vi "RTG Example.vi"() -> ()   [LabVIEW 2020, in "RTG Examples.lvlib"]
doc: "This example illustrates how to use the RTG local API to control the RTG."
uses:
  RTG Examples.lvlib
  <vilib>/RTG/API/ip/common/host-types/Target Configuration.ctl
  <vilib>/RTG/API/ip/common/host-types/Synchronization - Host.ctl
  <vilib>/RTG/API/ip/common/host-types/Synchronization Mode - Host.ctl
  <vilib>/RTG/API/ip/common/host-types/Basic Target - Host.ctl
  <vilib>/RTG/API/interface/public/State.ctl
  <vilib>/RTG/coprocessor/host/RTG Coprocessor Link Interface/Public/Coprocessor Status.ctl
  <vilib>/RTG/API/ip/common/host-types/Target Motion Parameters.ctl
  <vilib>/RTG/API/ip/common/host-types/Single Target Motion Parameters.ctl
  support/Options - API Mode.ctl
  support/Options - Calibration.ctl
  support/Options - Remote.ctl
  <vilib>/RTG/API/interface/public/Coprocessor Link Status.ctl
  <vilib>/Utility/error.llb/Error Cluster From Error Code.vi
  <vilib>/rvi/errors/niLvFpgaAdjustHostInterfaceError.vi
  <vilib>/rvi/interface/nirviReadWriteControl/nirviReadWriteControl.xnode
  <vilib>/RTG/API/interface/NI-RTG Interface.lvclass
  <vilib>/RTG/coprocessor/host/RTG Coprocessor Link Interface/RTG Coprocessor Link Interface.lvclass
  <vilib>/RTG/API/ip/common/host-types/Host Data Types v1.lvlib
  NiFpgaLv.dll
  <vilib>/rvi/interface/Simulation/niFpgaSimulationCallBeginRW.vi
panel:
  out "Bitfiles Loaded":bool
  out "RTG Status":string
  out "RTG State":T1
  in  "tab":T2(tab)
  in  "abort system self cal":bool
  in  "Set PRIs":bool
  in  "PRI (s)":dbl[](array[numeric]) format="%#_6p"
  in  "Calibrate":bool=TRUE
  in  "Instrument Names":string[](array[string])=["5831_0"]
  in  "Center Freqeuncies (Hz)":dbl[](array[numeric])=[5500000000.0] format="%#_6p"
  in  "Reference Levels (dBm)":dbl[](array[numeric])=[0.0]
  in  "mmWave Radio Heads Enable":bool[](array[boolean])
  in  "External Delay (s)":dbl[](array[numeric]) format="%#_6p"
  in  "External Attenuations (dB)":dbl[](array[numeric])
  in  "Offset Frequencies (Hz)":dbl[](array[numeric]) format="%#_6p"
  out "Error Out":errorcluster caption="error out"
  in  "RTG API Options":T6={"API Mode"=enum."Local", "Calibration Options"={"enable internal loopback  "=FALSE, "enable overwrite cal data  "=FALSE, "enable save cal data           "=FALSE, "disable self cal range          "=FALSE}, "Remote Options"={"ip address"="", "port"="50052", "certificate path"=path "", "timeout (ms)"=15000}, "ini file path"=path ""}
  in  "Option String Override":string
  in  "Coprocessor Names":string[](array[string])
  out "Versions":string[](array[string])
  out "Max Common Attenuations (dB)":dbl[](array[numeric])
  out "Min Common Attenuations (dB)":dbl[](array[numeric])
  out "Min Latencies (s)":dbl[](array[numeric]) format="%#_6p"
  in  "configure common attenuation":bool
  in  "Common Attenuation (dB)":dbl
  in  "set hardware trigger":bool
  in  "send target motion":bool
  in  "Auto Send Software Trigger":bool
  in  "Prepend Software Trigger":bool
  in  "send files":bool
  in  "Target Configuration Files":path[](array[path])
  in  "pulse detection calibration":bool
  in  "send target config":bool
  in  "send sw trigger":bool
  in  "start rtg":bool
  in  "stop rtg":bool
  in  "abort":bool
  in  "Target Configuration":T7 {"rtg targets"."time offset (s)" format="%#_6p"; "rtg targets"."doppler" format="%#_6p"}
  in  "Device Index":i32
  in  "Target Motion Parameters":T11={"target motions"=[{"target enable"=FALSE, "start time offset (s)"=-1e-09, "time offset rate of change (s/s)"=0.001, "start attenuation (dB)"=0.0, "attenuation rate of change (dB/s)"=0.0, "start frequency shift (Hz)"=0.0, "frequency shift rate of change (Hz/sec)"=0.0}], "scenario duration (s)"=67.0, "configuration update rate(Hz)"=15000.0} {"configuration update rate(Hz)" format="%#_6p"; "target motions"."frequency shift rate of change (Hz/sec)" format="%#_6p"; "target motions"."start frequency shift (Hz)" format="%#_6p"; "target motions"."time offset rate of change (s/s)" format="%#_6p"; "target motions"."start time offset (s)" format="%#_6p"}
  in  "Data Path Enable":bool=TRUE
  in  "Hardware Trigger":string="PXI_Trig7"
  out "Device Index vs Trigger Count":i32[][](array[numeric])
  out "coprocessor link status":T13[](array[typedef])
  out "rtg link status":T14[](array[typedef])
  # "Coprocessor"
  # "Configuration Files and Target Motion"
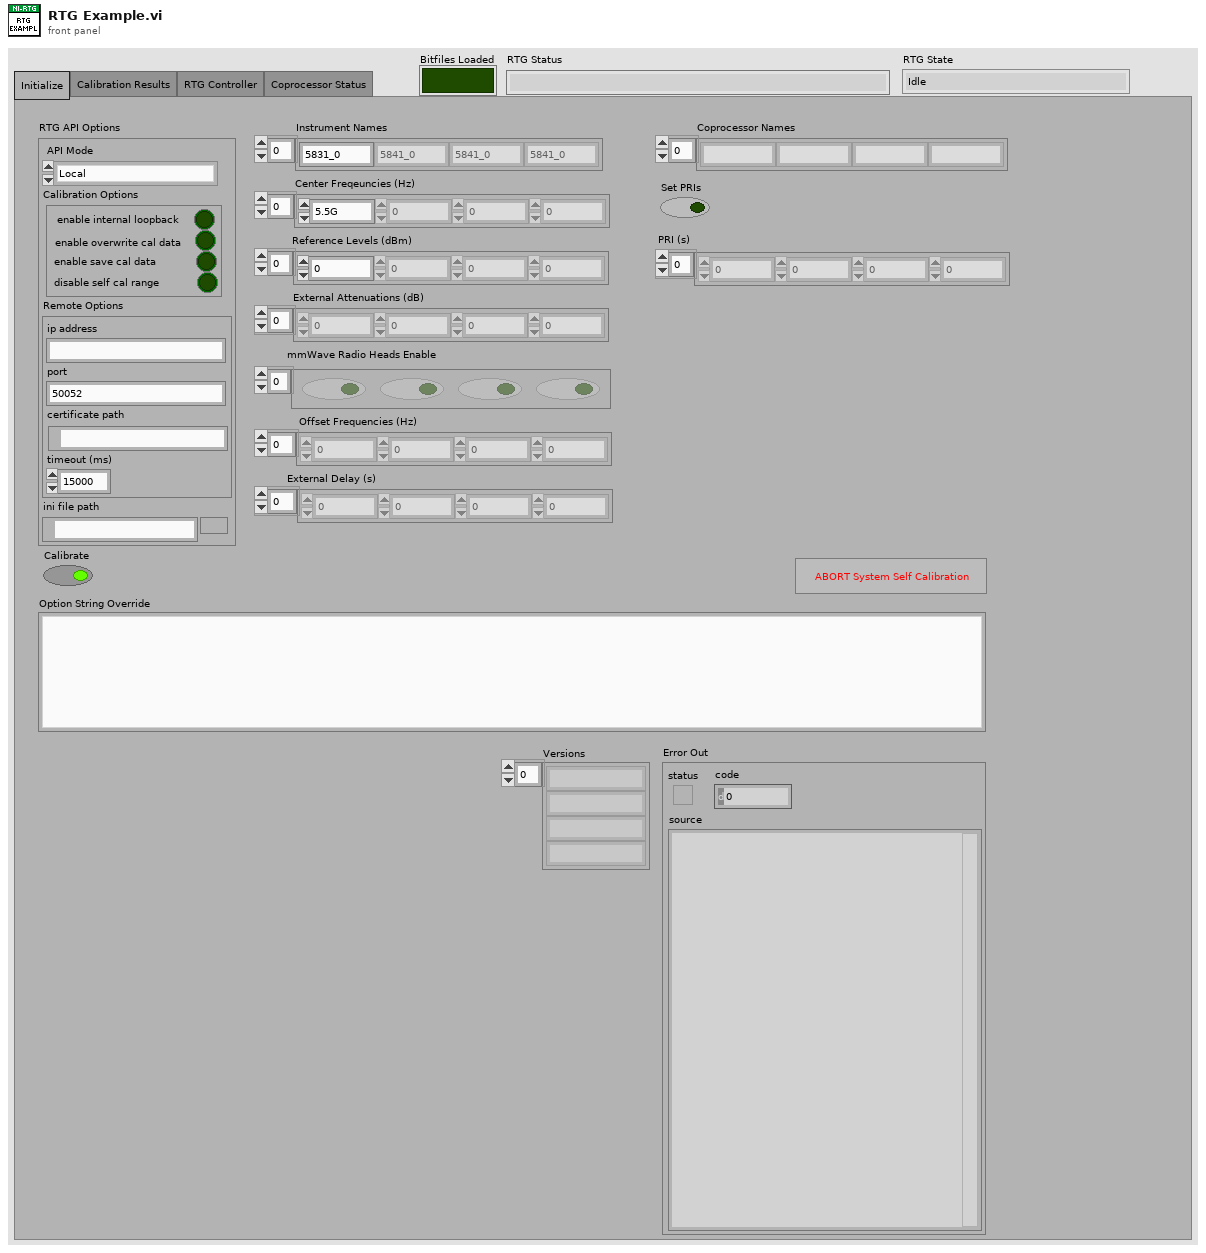
[diagram p1: front panel]
types:
  T1 = typedef "NI-RTG v1.lvlib/NI-RTG Interface.lvclass/State.ctl" = enum16{"Idle", "Inactive", "Active", "System Self Calibration"}
  T2 = enum32{"Initialize", "Calibration Results", "RTG Controller", "Coprocessor Status"}
  T3 = typedef "RTG Examples.lvlib/Options - API Mode.ctl" = enum16{"Local", "Remote"}
  T4 = typedef "RTG Examples.lvlib/Options - Calibration.ctl" = cluster{"enable internal loopback  ":bool, "enable overwrite cal data  ":bool, "enable save cal data           ":bool, "disable self cal range          ":bool}
  T5 = typedef "RTG Examples.lvlib/Options - Remote.ctl" = cluster{"ip address":string, "port":string, "certificate path":path, "timeout (ms)":i32}
  T6 = cluster{"API Mode":T3, "Calibration Options":T4, "Remote Options":T5, "ini file path":path}
  T7 = typedef "Host Data Types v1.lvlib/Target Configuration.ctl" = cluster{"synchronization":T8, "rtg targets":T10[]}
  T8 = typedef "Host Data Types v1.lvlib/Synchronization - Host.ctl" = cluster{"synch mode":T9, "time offset (s)":dbl}
  T9 = typedef "Host Data Types v1.lvlib/Synchronization Mode - Host.ctl" = enum16{"Software Trigger", "Hardware Trigger", "Time Offset Relative to First", "Time Offset Relative to Last", "Pulse Rising Edge", "Pulse Falling Edge"}
  T10 = typedef "Host Data Types v1.lvlib/Basic Target - Host.ctl" = cluster{"time offset (s)":dbl, "attenuaton (dB)":dbl, "doppler":dbl, "target enable":bool, "relative velocity enable":bool}
  T11 = typedef "Host Data Types v1.lvlib/Target Motion Parameters.ctl" = cluster{"target motions":T12[], "scenario duration (s)":dbl, "configuration update rate(Hz)":dbl}
  T12 = typedef "Host Data Types v1.lvlib/Single Target Motion Parameters.ctl" = cluster{"target enable":bool, "start time offset (s)":dbl, "time offset rate of change (s/s)":dbl, "start attenuation (dB)":dbl, "attenuation rate of change (dB/s)":dbl, "start frequency shift (Hz)":dbl, "frequency shift rate of change (Hz/sec)":dbl}
  T13 = typedef "RTG Coprocessor Link Interface v1 Host.lvlib/RTG Coprocessor Link Interface.lvclass/Coprocessor Status.ctl" = cluster{"tx read count":u64, "tx read overflow":bool, "rx read count":u64, "rx read overflow":bool}
  T14 = typedef "NI-RTG v1.lvlib/NI-RTG Interface.lvclass/Coprocessor Link Status.ctl" = cluster{"task name":string, "device name":string, "hard error":bool, "soft error":bool, "channel up":bool, "system reset":bool}
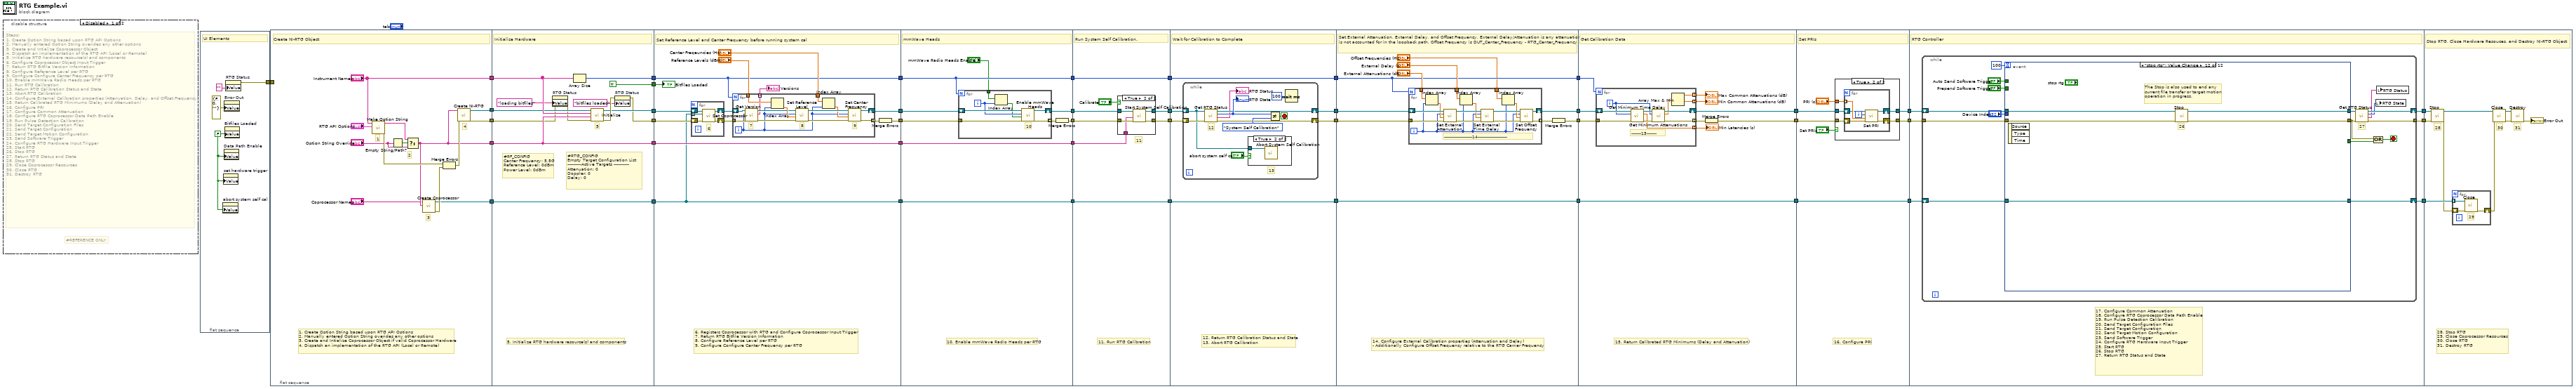
[diagram p0: block diagram]
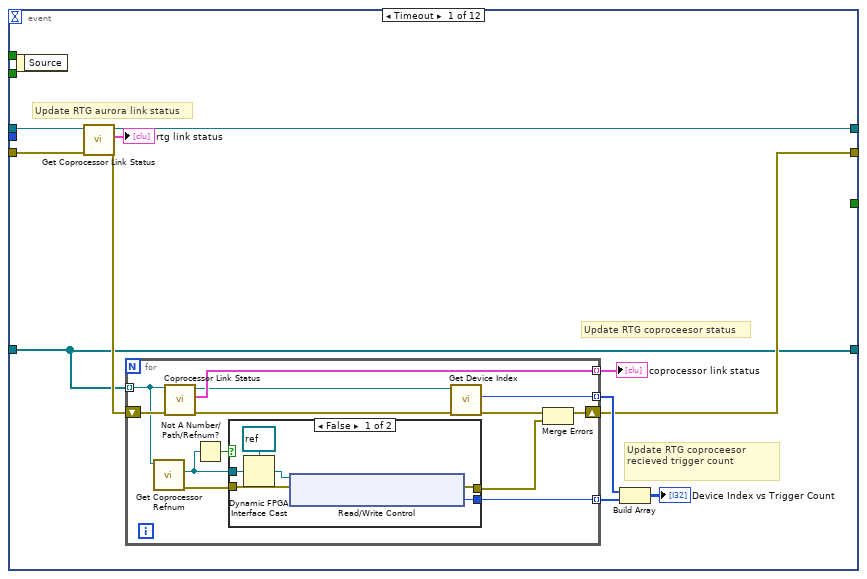
[diagram p6: hidden frame]
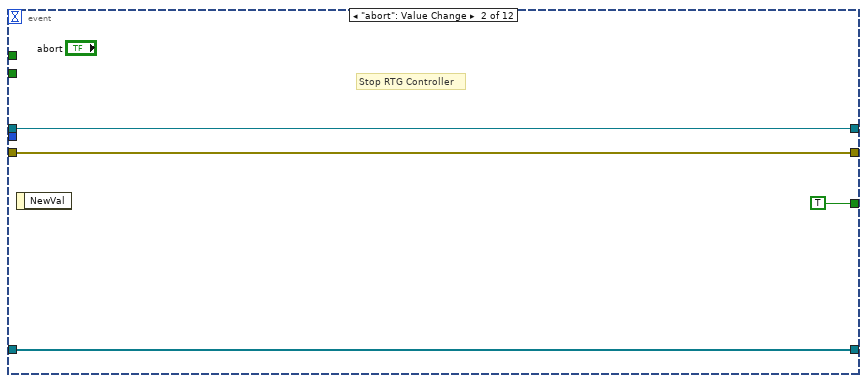
[diagram p8: hidden frame]
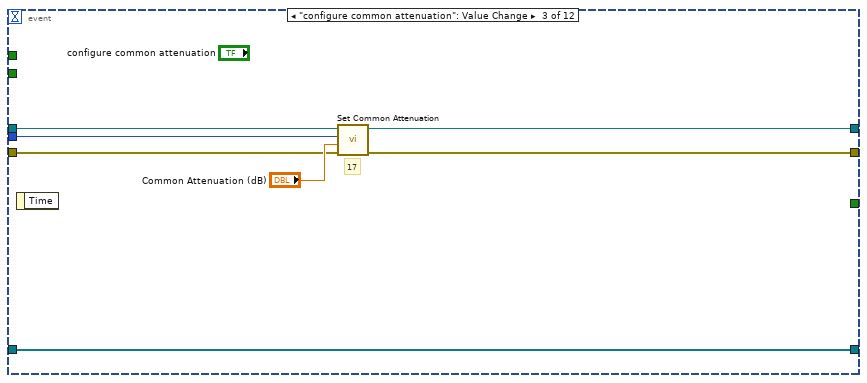
[diagram p9: hidden frame]
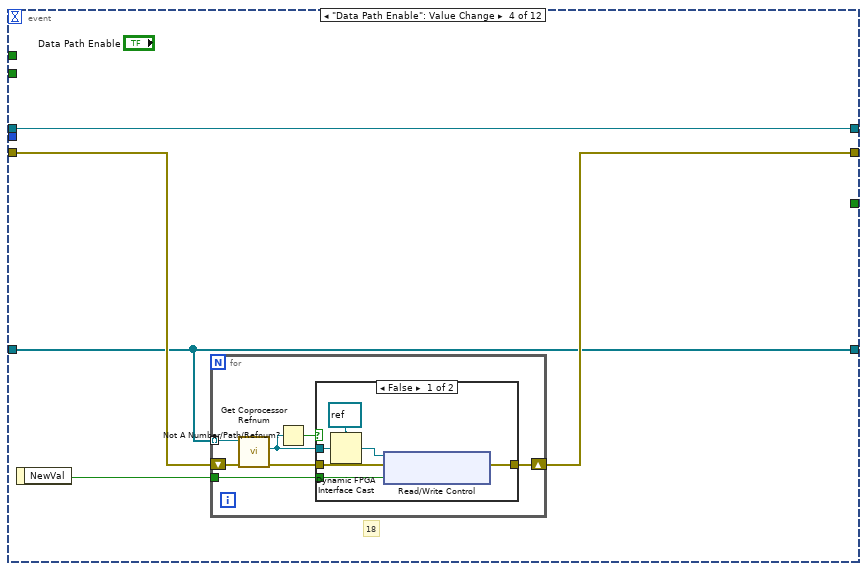
[diagram p10: hidden frame]
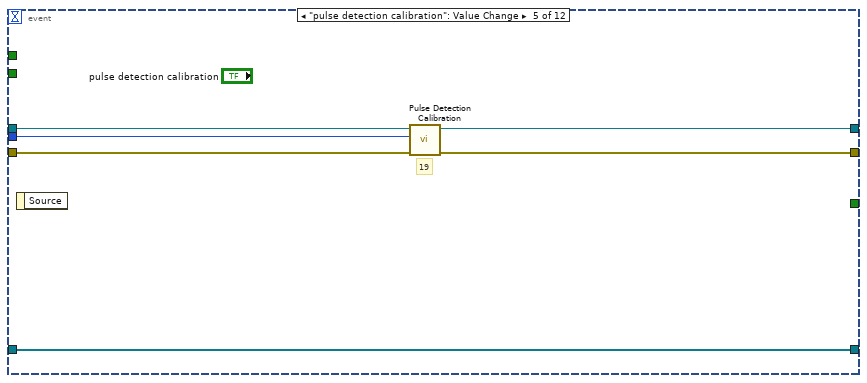
[diagram p12: hidden frame]
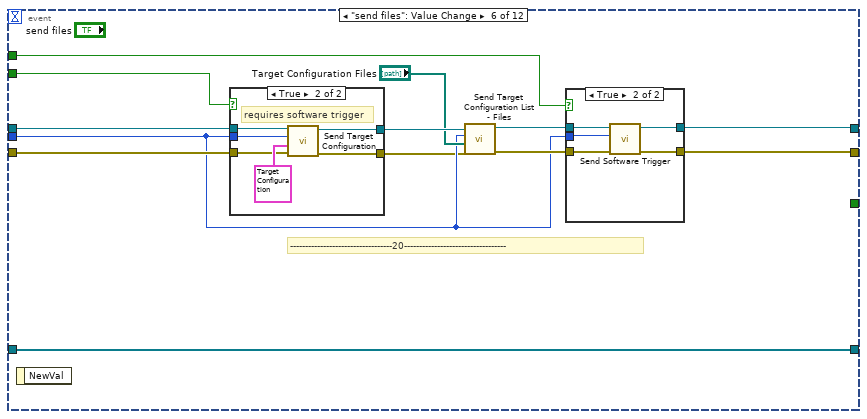
[diagram p13: hidden frame]
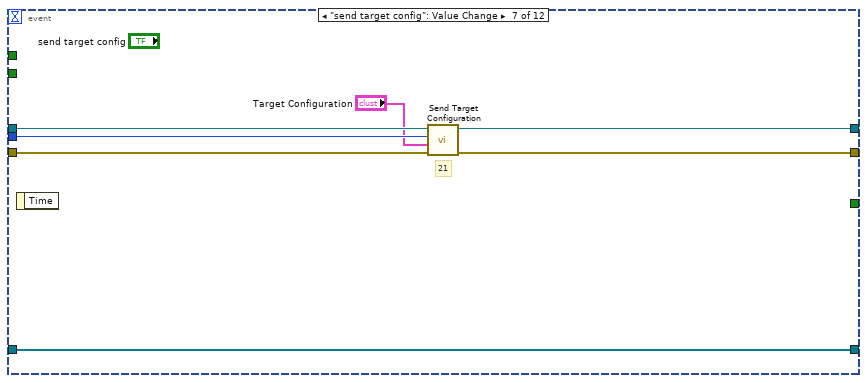
[diagram p16: hidden frame]
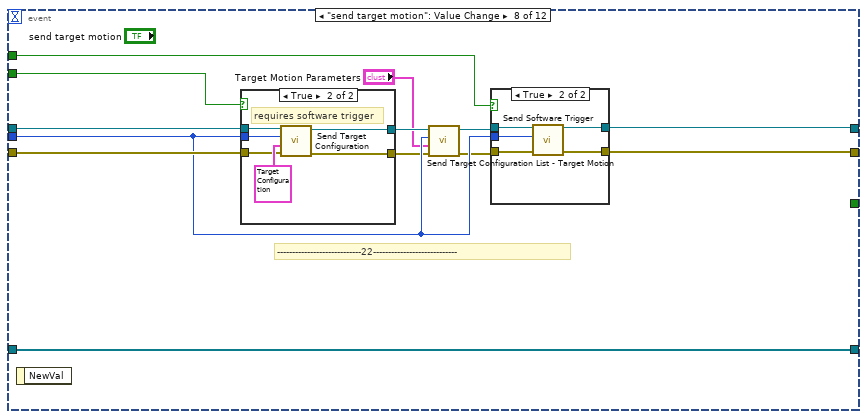
[diagram p17: hidden frame]
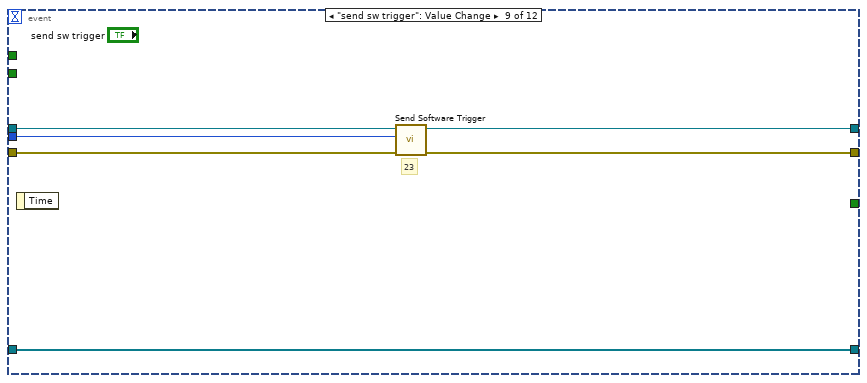
[diagram p20: hidden frame]
diagram:
  n1 = disable-structure shown="Disabled" {
    frame Disabled {
      # "#REFERENCE ONLY"
      # "Steps:\n1. Create Option String based upon RTG API Options\n2. Manually entered Option String overides any other options\n3. Create and Intialize Coprocessor Object\n4. Dispatch an implementation of the RTG API (Local or Remote)\n5. Initialize RTG hardware resource(s) and components\n6. Configure Coprocessor Object Input Trigger\n7. Return RTG Bitfile Version Information\n8. Configure Reference Level per RTG\n9. Configure Configure Center Frequency per RTG\n10. Enable mmWave Radio Heads per RTG\n11. Run RTG Calibration\n12. Return RTG Calibration Status and State\n13. Abort RTG Calibration\n14. Configure External Calibration properties (Attenuation, Delay, and Offset Frequency)\n15. Return Calibrated RTG Minimums (Delay and Attenuation)\n16. Configure PRI\n17. Configure Common Attenuation\n18. Configure RTG Coprocessor Data Path Enable \n19. Run Pulse Detection Calibration\n20. Send Target Configuration Files\n21. Send Target Configuration\n22. Send Target Motion Configuration\n23. Send Software Trigger\n24. Configure RTG Hardware Input Trigger\n25. Start RTG\n26. Stop RTG\n27. Return RTG Status and State\n28. Stop RTG\n29. Close Coprocessor Resources\n30. Close RTG\n31. Destroy RTG"
    }
    frame Enabled {
    }
  }
  n2 = flat-sequence {
    tunnel: [w46] -> w8
    frame #0 {
      w44 = FALSE ("bitfiles loaded")
      # "UI Elements"
      n3 = property on="abort system self cal" class="Bool (strict)"("Value"=w44) -> ()  [unwired: 2 in, 2 out]
      n4 = property on="set hardware trigger" class="Bool (strict)"("Value"=w44) -> ()  [unwired: 2 in, 2 out]
      n5 = property on="Data Path Enable" class="Bool (strict)"("Value"=w44) -> ()  [unwired: 2 in, 2 out]
      n6 = property on="Error Out" class="Clust (strict)"("Value"=errorcluster {"status"=FALSE, "code"=0, "source"=""} ("error out")) -> ()  [unwired: 2 in, 2 out]
      n7 = property on="Bitfiles Loaded" class="Bool (strict)"("Value"=w44) -> ()  [unwired: 2 in, 2 out]
      n8 = property on="RTG Status" class="Str"("Value"="" ("rtg status")) -> (error out=w46:errorcluster)  [unwired: 2 in, 1 out]
    }
  }
  n9 = flat-sequence {
    tunnel: [w60] -> w29
    tunnel: [w49] -> w28
    tunnel: ["Instrument Names"] -> w18
    tunnel: [w59] -> w17
    tunnel: [w52] -> w16
    tunnel: w8 -> [_]
    tunnel: [w61] -> w43
    tunnel: [w62] -> w42
    tunnel: [w73] -> w41
    tunnel: w29 -> [w69]
    tunnel: w28 -> [w71]
    tunnel: [w71] -> w21
    tunnel: w18 -> [w72]
    tunnel: w17 -> [w65]
    tunnel: w16 -> [w70]
    tunnel: [w70] -> w15
    tunnel: [TRUE] -> w7
    tunnel: w43 -> [w78]
    tunnel: w42 -> [w74]
    tunnel: [w85] -> w35
    tunnel: [w83] -> w33
    tunnel: w41 -> [w82]
    tunnel: [w82] -> w31
    tunnel: w21 -> [w81]
    tunnel: [w81] -> w20
    tunnel: w15 -> [w77]
    tunnel: [w77] -> w13
    tunnel: w7 -> [w76]
    tunnel: w35 -> [w114]
    tunnel: [w109] -> w34
    tunnel: w33 -> [w113]
    tunnel: [w111] -> w32
    tunnel: w31 -> [w115]
    tunnel: [w115] -> w30
    tunnel: w20 -> [w108]
    tunnel: [w108] -> w19
    tunnel: [w107] -> w14
    tunnel: w13 -> [w107]
    tunnel: w34 -> [w130]
    tunnel: w32 -> [w129]
    tunnel: [w127] -> w27
    tunnel: [w128] -> w26
    tunnel: w30 -> [w128]
    tunnel: [w126] -> w24
    tunnel: w19 -> [w125]
    tunnel: w14 -> [w123]
    tunnel: [w123] -> w12
    tunnel: w27 -> [w142]
    tunnel: w26 -> [w143]
    tunnel: [w143] -> w25
    tunnel: w24 -> [w141]
    tunnel: [w140] -> w23
    tunnel: [w139] -> w22
    tunnel: w12 -> [w138]
    tunnel: [w138] -> w11
    tunnel: [w161] -> w38
    tunnel: [w160] -> w37
    tunnel: [w159] -> w36
    tunnel: w25 -> [w159]
    tunnel: w23 -> [w158]
    tunnel: w22 -> [w157]
    tunnel: w11 -> [w155]
    tunnel: [w155] -> w10
    tunnel: w38 -> [w187]
    tunnel: [w186] -> w6
    tunnel: w37 -> [w189]
    tunnel: [w185] -> w4
    tunnel: w36 -> [w181]
    tunnel: w10 -> [w180]
    tunnel: [w180] -> w2
    tunnel: w6 -> [w205]
    tunnel: [w204] -> w5
    tunnel: w4 -> [w203]
    tunnel: [w202] -> w3
    tunnel: w2 -> [w207]
    tunnel: [w207] -> w1
    tunnel: w5 -> [w226]
    tunnel: w3 -> [w225]
    tunnel: [w224] -> w40
    tunnel: [w223] -> w39
    tunnel: w1 -> [w222]
    tunnel: [w221] -> w9
    tunnel: w40 -> [w415]
    tunnel: w39 -> [w409]
    tunnel: w9 -> [w410]
    frame #0 {
      # "1. Create Option String based upon RTG API Options\n2. Manually entered Option String overides any other options\n3. Create and Intialize Coprocessor Object if valid Coprocessor Hardware\n4. Dispatch an implementation of the RTG API (Local or Remote)"
      # "4"
      # "3"
      # "2"
      # "1"
      # "Create NI-RTG Object"
      n10 = call "Make Option String.vi"("rtg api options"="RTG API Options", "instrument names"="Instrument Names") -> ("error out"=w53:errorcluster, "option string"=w55:string)  [unwired: 8 in]
      n11 = Empty String/Path?(string/path="Option String Override") -> (empty?=w56:bool)
      n12 = Select(t=w55, s=w56, f="Option String Override") -> (s? t:f=w49:string)
      n13 = call <vilib>:"Create Coprocessor.vi"("option string"=w49, "coprocessor resources"="Coprocessor Names") -> ("error out"=w54:errorcluster, "rtg coprocessor links"=w52:refnum<class "RTG Coprocessor Link Interface.lvclass">[])  [unwired: 8 in]
      n14 = Merge Errors(w53, w54) -> (w58:errorcluster)
      n15 = call <vilib>:"Create NI-RTG.vi"("error in"=w58, "option string"=w49) -> ("error out"=w59:errorcluster, "NI-RTG Interface out"=w60:refnum<class "NI-RTG Interface.lvclass">)  [unwired: 8 in]
    }
    frame #1 {
      # "5. Initialize RTG hardware resource(s) and components"
      # "5"
      # "#RTG_CONFIG\nEmpty Target Configuration List\n----------Active Targets -----------\nAttenuation: 0\nDoppler: 0\nDelay: 0"
      # "#RF_CONFIG\nCenter Frequency: 5.5G\nReference Level: 0dBm\nPower Level: 0dBm"
      # "Initialize Hardware"
      n16 = property on="RTG Status" class="Str"(error in=w65, "Value"="loading bitfiles" ("rtg status")) -> (error out=w64:errorcluster)  [unwired: 1 in, 1 out]
      n17 = Array Size(array=w72) -> (size(s)=w73:i32)
      n18 = call-dynamic "Initialize.vi"("error in"=w64, "option string"=w71, "instrument names"=w72, "ni-rtg interface"=w69) -> ("error out"=w68:errorcluster, "ni-rtg interface out"=w62:refnum<class "NI-RTG Interface.lvclass">)  [unwired: 6 in]
      n19 = property on="RTG Status" class="Str"(error in=w68, "Value"="bitfiles loaded" ("rtg status")) -> (error out=w61:errorcluster)  [unwired: 1 in, 1 out]
    }
    frame #2 {
      # "6. Registers Coprocessor with RTG and Configure Coprocessor Input Trigger\n7. Return RTG Bitfile Version Information\n8. Configure Reference Level per RTG\n9. Configure Configure Center Frequency per RTG"
      # "Set Reference Level and Center Frequency before running system cal"
      n20 = for {
        shift-right: [w106] -> w80
        shift-left: w78 -> [w104]
        shift-right: [w105] -> w79
        shift-left: w74 -> [w103]
        tunnel: w77 -> [w102] mode=indexing
        # "6"
        n21 = call-dynamic "Set Coprocessor.vi"("error in"=w104, "rtg coprocessor link interface"=w102, "rtg api interface"=w103) -> ("error out"=w106:errorcluster, "rtg api interface out"=w105:refnum<class "NI-RTG Interface.lvclass">)  [unwired: 7 in]
      }
      n22 = for {
        N: w82 -> [_]
        tunnel: w80 -> [w91]
        tunnel: "Reference Levels (dBm)" -> [w99]
        tunnel: "Center Freqeuncies (Hz)" -> [w97]
        shift-right: [w95] -> w85
        shift-left: w79 -> [w93]
        tunnel: [w94] -> w84 mode=indexing
        tunnel: [w88] -> w75 mode=indexing
        i -> [w89]
        # "9"
        # "8"
        # "7"
        n23 = call-dynamic "Get Version.vi"("error in"=w91, "device index (0)"=w89, "NI-RTG Interface in"=w93) -> ("error out"=w90:errorcluster, "version"=w88:string, "NI-RTG Interface out"=w92:refnum<class "NI-RTG Interface.lvclass">)  [unwired: 6 in]
        n24 = Index Array(array=w99, index=w89) -> (element=w98:dbl)
        n25 = call-dynamic "Set Reference Level.vi"("error in"=w90, "reference level (dBm)"=w98, "device index (0)"=w89, "rtg api interface"=w92) -> ("error out"=w100:errorcluster, "rtg api interface out"=w101:refnum<class "NI-RTG Interface.lvclass">)  [unwired: 6 in]
        n26 = Index Array(array=w97, index=w89) -> (element=w96:dbl)
        n27 = call-dynamic "Set Center Frequency.vi"("error in"=w100, "center frequency (Hz)"=w96, "device index (0)"=w89, "rtg api interface"=w101) -> ("error out"=w94:errorcluster, "rtg api interface out"=w95:refnum<class "NI-RTG Interface.lvclass">)  [unwired: 6 in]
      }
      "Versions" <- w75
      n28 = Merge Errors(w84) -> (w83:errorcluster)
      "Bitfiles Loaded" <- w76
    }
    frame #3 {
      # "10. Enable mmWave Radio Heads per RTG"
      # "mmWave Heads"
      n29 = for {
        N: w115 -> [_]
        shift-right: [w119] -> w109
        shift-left: w114 -> [w120]
        tunnel: w113 -> [w122]
        tunnel: [w121] -> w112 mode=indexing
        tunnel: "mmWave Radio Heads Enable" -> [w118]
        i -> [w117]
        # "10"
        n30 = Index Array(array=w118, index=w117) -> (element=w116:bool)
        n31 = call-dynamic "Enable mmWave Heads.vi"("error in"=w122, "enable mmWave"=w116, "device index (0)"=w117, "ni-rtg interface"=w120) -> ("error out"=w121:errorcluster, "ni-rtg interface out"=w119:refnum<class "NI-RTG Interface.lvclass">)  [unwired: 6 in]
      }
      n32 = Merge Errors(w112) -> (w111:errorcluster)
    }
    frame #4 {
      # "11. Run RTG Calibration"
      # "11"
      # "Run System Self Calibration."
      n33 = case shown="True" "Calibrate" {
        tunnel: w130 -> [w132 w137]
        tunnel: w129 -> [w131 w136]
        tunnel: [w132 w135] -> w127
        tunnel: [w131 w134] -> w126
        tunnel: w125 -> [_ w133]
        frame False {
        }
        frame True {
          n34 = call-dynamic "Start System Self Calibration.vi"("error in"=w136, "option string"=w133, "rtg api interface"=w137) -> ("error out"=w134:errorcluster, "rtg api interface out"=w135:refnum<class "NI-RTG Interface.lvclass">)  [unwired: 7 in]
        }
      }
    }
    frame #5 {
      # "12. Return RTG Calibration Status and State\n13. Abort RTG Calibration"
      # "Wait for Calibration to Complete"
      n35 = while {
        shift-right: [w149] -> w140
        shift-left: w142 -> [w145]
        shift-right: [w150] -> w139
        shift-left: w141 -> [w153]
        stop <- w148 stop-if-true
        # "13"
        # "12"
        n36 = call-dynamic "Get RTG Status.vi"("error in"=w153, "rtg api interface"=w145) -> ("error out"=w150:errorcluster, "rtg status"=→"RTG Status":string, "state"=w152:T1, "rtg api interface out"=w149:refnum<class "NI-RTG Interface.lvclass">)  [unwired: 6 in]
        "RTG State" <- w152
        n37 = case shown="True" "abort system self cal" {
          tunnel: w145 -> [_ w154]
          frame False {
          }
          frame True {
            n38 = call-dynamic "Abort System Self Calibration.vi"("rtg-api interface"=w154) -> ()  [unwired: 9 in, 2 out]
          }
        }
        n39 = Not Equal?(x=w152, y=State."System Self Calibration") -> (x != y?=w148:bool)
        n40 = Wait (ms)(milliseconds to wait=u32 100) -> ()  [unwired: 1 out]
      }
    }
    frame #6 {
      # "14. Configure External Calibration properties (Attenuation and Delay)\n- Additionally Configure Offset Frequency relative to the RTG Carrier Frequency"
      # "Set External Attenuation, External Delay, and Offset Frequency. External Delay/Attenuation is any attenuation/delay that is not accounted for in the loopback path. Offset Frequency is DUT_Center_Frequency - RTG_Center_Frequency"
      n41 = for {
        N: w159 -> [_]
        shift-right: [w169] -> w161
        shift-left: w158 -> [w179]
        tunnel: "External Attenuations (dB)" -> [w177]
        tunnel: "External Delay (s)" -> [w175]
        tunnel: [w171] -> w162 mode=indexing
        tunnel: w157 -> [w168]
        tunnel: "Offset Frequencies (Hz)" -> [w167]
        i -> [w165]
        # "--------------------14---------------------"
        n42 = Index Array(array=w177, index=w165) -> (element=w176:dbl)
        n43 = call-dynamic "Set External Attenuation.vi"("error in"=w168, "external attenuation (dB)"=w176, "device index (0)"=w165, "rtg api interface"=w179) -> ("error out"=w173:errorcluster, "rtg api interface out"=w178:refnum<class "NI-RTG Interface.lvclass">)  [unwired: 6 in]
        n44 = Index Array(array=w175, index=w165) -> (element=w174:dbl)
        n45 = call-dynamic "Set External Time Delay.vi"("error in"=w173, "delay (s)"=w174, "device index (0)"=w165, "rtg api interface"=w178) -> ("error out"=w172:errorcluster, "rtg api interface out"=w170:refnum<class "NI-RTG Interface.lvclass">)  [unwired: 6 in]
        n46 = Index Array(array=w167, index=w165) -> (element=w166:dbl)
        n47 = call-dynamic "Set Offset Frequency.vi"("error in"=w172, "offset frequency (Hz)"=w166, "device index (0)"=w165, "NI-RTG Interface in"=w170) -> ("error out"=w171:errorcluster, "NI-RTG Interface out"=w169:refnum<class "NI-RTG Interface.lvclass">)  [unwired: 6 in]
      }
      n48 = Merge Errors(w162) -> (w160:errorcluster)
    }
    frame #7 {
      # "15. Return Calibrated RTG Minimums (Delay and Attenuation)"
      # "Get Calibration Data"
      n49 = for {
        N: w181 -> [_]
        tunnel: w189 -> [w200]
        tunnel: [w197] -> w188 mode=indexing
        shift-right: [w195] -> w186
        shift-left: w187 -> [w198]
        tunnel: [w194] -> w182 mode=indexing
        tunnel: [w192] -> w184 mode=indexing
        tunnel: [w191] -> w183 mode=indexing
        i -> [w190]
        # "-------15-------"
        n50 = call-dynamic "Get Minimum Time Delay.vi"("error in"=w200, "device index (0)"=w190, "rtg api interface"=w198) -> ("error out"=w199:errorcluster, "delay (s)"=w194:dbl, "rtg api interface out"=w196:refnum<class "NI-RTG Interface.lvclass">)  [unwired: 5 in, 1 out]
        n51 = call-dynamic "Get Minimum Attenuations.vi"("error in"=w199, "device index (0)"=w190, "rtg api interface"=w196) -> ("error out"=w197:errorcluster, "attenuations (dB)"=w193:dbl[], "rtg api interface out"=w195:refnum<class "NI-RTG Interface.lvclass">)  [unwired: 5 in, 1 out]
        n52 = Array Max & Min(array=w193) -> (max value=w192:dbl, min value=w191:dbl)  [unwired: 2 out]
      }
      "Max Common Attenuations (dB)" <- w184
      "Min Common Attenuations (dB)" <- w183
      "Min Latencies (s)" <- w182
      n53 = Merge Errors(w188) -> (w185:errorcluster)
    }
    frame #8 {
      # "16. Configure PRI"
      # "Set PRIs"
      n54 = case shown="True" "Set PRIs" {
        tunnel: w205 -> [w209 w211]
        tunnel: [w209 w213] -> w204
        tunnel: w203 -> [w208 w210]
        tunnel: [w208 w212] -> w202
        tunnel: "PRI (s)" -> [_ w214]
        frame False {
        }
        frame True {
          n55 = for {
            tunnel: w214 -> [w220] mode=indexing
            shift-right: [w218] -> w213
            shift-left: w211 -> [w216]
            shift-right: [w217] -> w212
            shift-left: w210 -> [w215]
            i -> [w219]
            n56 = call-dynamic "Set PRI.vi"("error in"=w215, "pri (s)"=w220, "device index (0)"=w219, "NI-RTG Interface in"=w216) -> ("error out"=w217:errorcluster, "NI-RTG Interface out"=w218:refnum<class "NI-RTG Interface.lvclass">)  [unwired: 6 in]
          }
        }
      }
    }
    frame #9 {
      # "17. Configure Common Attenuation\n18. Configure RTG Coprocessor Data Path Enable \n19. Run Pulse Detection Calibration\n20. Send Target Configuration Files\n21. Send Target Configuration\n22. Send Target Motion Configuration\n23. Send Software Trigger\n24. Configure RTG Hardware Input Trigger\n25. Start RTG\n26. Stop RTG\n27. Return RTG Status and State"
      # "RTG Controller"
      n57 = while {
        tunnel: w225 -> [w241]
        shift-right: [w237] -> w224
        shift-left: w226 -> [w242]
        tunnel: [w236] -> w223
        shift-right: [w232] -> w221
        shift-left: w222 -> [w233]
        stop <- w230 stop-if-true
        # "27"
        n58 = event shown="[11] \"stop rtg\": Value Change" {
          selector: _ -> [_ _ _ _ _ _ _ _ _ _ _ _]
          dyn-events: _ -> [_ _ _ _ _ _ _ _ _ _ _ _]
          timeout: 100 -> [_ _ _ _ _ _ _ _ _ _ _ _]
          tunnel: [_ TRUE _ _ _ _ _ _ _ _ _ _] -> w240
          tunnel: w242 -> [w253 w276 w284 w289 w307 w321 w344 w356 w378 w384 w401 w406]
          tunnel: w241 -> [w245 w275 w279 w287 w305 w320 w339 w355 w374 w383 w398 w403]
          tunnel: [w252 w276 w283 w289 w308 w316 w343 w354 w377 w385 w400 w405] -> w238
          tunnel: [w244 w275 w278 w286 w304 w312 w338 w347 w373 w379 w397 w402] -> w229
          tunnel: "Device Index" -> [_ _ w282 _ w309 w314 w342 w353 w376 w382 _ _]
          tunnel: w233 -> [w243 w274 w280 w285 w306 w322 w340 w357 w375 w380 w399 w404]
          tunnel: [w243 w274 w280 w285 w306 w322 w340 w357 w375 w380 w399 w404] -> w232
          tunnel: "Auto Send Software Trigger" -> [_ _ _ _ _ w311 _ w345 _ _ _ _]
          tunnel: "Prepend Software Trigger" -> [_ _ _ _ _ w310 _ w346 _ _ _ _]
          event Timeout {
            # "Update RTG coproceesor \nrecieved trigger count"
            # "Update RTG coproceesor status"
            # "Update RTG aurora link status"
            n59 = event-data() -> ()  [unwired: 1 in, 1 out]
            n60 = call-dynamic "Get Coprocessor Link Status.vi"("error in"=w245, "rtg api interface"=w253) -> ("error out"=w251:errorcluster, "rtg link status"=→"rtg link status":T14[], "rtg api interface out"=w252:refnum<class "NI-RTG Interface.lvclass">)  [unwired: 7 in]
            n61 = for {
              tunnel: w243 -> [w261] mode=indexing
              tunnel: [w265] -> w250 mode=indexing
              shift-right: [w258] -> w244
              shift-left: w251 -> [w266]
              tunnel: [w260] -> w248 mode=indexing
              tunnel: [w254] -> w249 mode=indexing
              n62 = call-dynamic "Get Coprocessor Refnum.vi"("rtg coprocessor link interface"=w261) -> ("error out"=w264:errorcluster, "coprocessor refnum"=w262:refnum<k20>)  [unwired: 8 in, 1 out]
              n63 = call-dynamic "Coprocessor Link Status.vi"("error in"=w266, "rtg coprocessor link interface"=w261) -> ("error out"=w256:errorcluster, "coprocessor status out"=w265:T13, "rtg coprocessor link interface out"=w257:refnum<class "RTG Coprocessor Link Interface.lvclass">)  [unwired: 7 in]
              n64 = Not A Number/Path/Refnum?(number/path/refnum=w262) -> (NaN/Path/Refnum?=w263:bool)
              n65 = case shown="False" w263 {
                tunnel: w262 -> [w270 _]
                tunnel: w264 -> [w269 w273]
                tunnel: [w268 w273] -> w259
                tunnel: [w267 _] -> w260
                frame False {
                  n66 = Dynamic FPGA Interface Cast(Session In=refnum<k20> refnum ("Type"), Type=w270) -> (Session Out=w272:refnum<k20>)
                  n67 = xnode "Read/Write Control"("FPGA VI Reference In"=w272, "error in"=w269) -> ("error out"=w268:errorcluster, "read trigger rising edge count"=w267:u16)  [unwired: 1 out]
                }
                frame True {
                }
              }
              n68 = call-dynamic "Get Device Index.vi"("error in"=w256, "rtg coprocessor link interface"=w257) -> ("error out"=w255:errorcluster, "device index"=w254:i32)  [unwired: 7 in, 1 out]
              n69 = Merge Errors(w255, w259) -> (w258:errorcluster)
            }
            "coprocessor link status" <- w250
            n70 = Build Array(w249, w248) -> (→"Device Index vs Trigger Count":i32[][])
          }
          event "abort": Value Change {
            # "Stop RTG Controller"
            n71 = event-data() -> ()  [unwired: 1 in, 1 out]
          }
          event "configure common attenuation": Value Change {
            # "17"
            n72 = event-data() -> ()  [unwired: 1 in, 1 out]
            n73 = call-dynamic "Set Common Attenuation.vi"("error in"=w279, "attenuation (dB)"="Common Attenuation (dB)", "device index (0)"=w282, "rtg api interface"=w284) -> ("error out"=w278:errorcluster, "rtg api interface out"=w283:refnum<class "NI-RTG Interface.lvclass">)  [unwired: 5 in, 1 out]
          }
          event "Data Path Enable": Value Change {
            # "18"
            n74 = event-data() -> ("NewVal"=w288:bool)  [unwired: 1 in]
            n75 = for {
              tunnel: w285 -> [w296] mode=indexing
              tunnel: w288 -> [w293]
              shift-right: [w291] -> w286
              shift-left: w287 -> [w290]
              n76 = call-dynamic "Get Coprocessor Refnum.vi"("error in"=w290, "rtg coprocessor link interface"=w296) -> ("error out"=w292:errorcluster, "coprocessor refnum"=w295:refnum<k20>)  [unwired: 7 in, 1 out]
              n77 = Not A Number/Path/Refnum?(number/path/refnum=w295) -> (NaN/Path/Refnum?=w294:bool)
              n78 = case shown="False" w294 {
                tunnel: w295 -> [w300 _]
                tunnel: w293 -> [w299 _]
                tunnel: w292 -> [w298 w303]
                tunnel: [w297 w303] -> w291
                frame False {
                  n79 = Dynamic FPGA Interface Cast(Session In=refnum<k20> refnum ("Type"), Type=w300) -> (Session Out=w302:refnum<k20>)
                  n80 = xnode "Read/Write Control"("FPGA VI Reference In"=w302, "error in"=w298, "data path enable"=w299) -> ("error out"=w297:errorcluster)  [unwired: 1 out]
                }
                frame True {
                }
              }
            }
          }
          event "pulse detection calibration": Value Change {
            # "19"
            n81 = event-data() -> ()  [unwired: 1 in, 1 out]
            n82 = call-dynamic "Pulse Detection Calibration.vi"("error in"=w305, "device index (0)"=w309, "rtg api interface"=w307) -> ("error out"=w304:errorcluster, "rtg api interface out"=w308:refnum<class "NI-RTG Interface.lvclass">)  [unwired: 7 in]
          }
          event "send files": Value Change {
            # "----------------------------------20----------------------------------"
            n83 = event-data() -> ()  [unwired: 1 in, 1 out]
            n84 = case shown="True" w310 {
              tunnel: w321 -> [w331 w336]
              tunnel: w320 -> [w330 w333]
              tunnel: w314 -> [_ w335]
              tunnel: [w331 w334] -> w319
              tunnel: [w330 w332] -> w313
              frame False {
              }
              frame True {
                # "requires software trigger"
                n85 = call-dynamic "Send Target Configuration.vi"("error in"=w333, "target config"=T7 {"synchronization"={"synch mode"=enum."Software Trigger", "time offset (s)"=0.0}, "rtg targets"=[{"time offset (s)"=0.0, "attenuaton (dB)"=0.0, "doppler"=0.0, "target enable"=FALSE, "relative velocity enable"=FALSE}, {"time offset (s)"=0.0, "attenuaton (dB)"=0.0, "doppler"=0.0, "target enable"=FALSE, "relative velocity enable"=FALSE}, {"time offset (s)"=0.0, "attenuaton (dB)"=0.0, "doppler"=0.0, "target enable"=FALSE, "relative velocity enable"=FALSE}, {"time offset (s)"=0.0, "attenuaton (dB)"=0.0, "doppler"=0.0, "target enable"=FALSE, "relative velocity enable"=FALSE}]}, "device index (0)"=w335, "rtg api interface"=w336) -> ("error out"=w332:errorcluster, "rtg api interface out"=w334:refnum<class "NI-RTG Interface.lvclass">)  [unwired: 5 in, 1 out]
              }
            }
            n86 = call-dynamic "Send Target Configuration List - Files.vi"("error in"=w313, "target configuration file path"="Target Configuration Files", "device index (0)"=w314, "rtg api interface"=w319) -> ("error out"=w315:errorcluster, "rtg api interface out"=w317:refnum<class "NI-RTG Interface.lvclass">)  [unwired: 6 in]
            n87 = case shown="True" w311 {
              tunnel: w317 -> [w324 w329]
              tunnel: [w324 w328] -> w316
              tunnel: w315 -> [w323 w327]
              tunnel: [w323 w326] -> w312
              tunnel: w314 -> [_ w325]
              frame False {
              }
              frame True {
                n88 = call-dynamic "Send Software Trigger.vi"("error in"=w327, "device index (0)"=w325, "NI-RTG Interface in"=w329) -> ("error out"=w326:errorcluster, "NI-RTG Interface out"=w328:refnum<class "NI-RTG Interface.lvclass">)  [unwired: 7 in]
              }
            }
          }
          event "send target config": Value Change {
            # "21"
            n89 = event-data() -> ()  [unwired: 1 in, 1 out]
            n90 = call-dynamic "Send Target Configuration.vi"("error in"=w339, "target config"="Target Configuration", "device index (0)"=w342, "rtg api interface"=w344) -> ("error out"=w338:errorcluster, "rtg api interface out"=w343:refnum<class "NI-RTG Interface.lvclass">)  [unwired: 5 in, 1 out]
          }
          event "send target motion": Value Change {
            # "----------------------------22----------------------------"
            n91 = event-data() -> ()  [unwired: 1 in, 1 out]
            n92 = case shown="True" w346 {
              tunnel: w356 -> [w366 w371]
              tunnel: w355 -> [w365 w368]
              tunnel: w353 -> [_ w370]
              tunnel: [w366 w369] -> w352
              tunnel: [w365 w367] -> w348
              frame False {
              }
              frame True {
                # "requires software trigger"
                n93 = call-dynamic "Send Target Configuration.vi"("error in"=w368, "target config"=T7 {"synchronization"={"synch mode"=enum."Software Trigger", "time offset (s)"=0.0}, "rtg targets"=[{"time offset (s)"=0.0, "attenuaton (dB)"=0.0, "doppler"=0.0, "target enable"=FALSE, "relative velocity enable"=FALSE}, {"time offset (s)"=0.0, "attenuaton (dB)"=0.0, "doppler"=0.0, "target enable"=FALSE, "relative velocity enable"=FALSE}, {"time offset (s)"=0.0, "attenuaton (dB)"=0.0, "doppler"=0.0, "target enable"=FALSE, "relative velocity enable"=FALSE}, {"time offset (s)"=0.0, "attenuaton (dB)"=0.0, "doppler"=0.0, "target enable"=FALSE, "relative velocity enable"=FALSE}]}, "device index (0)"=w370, "rtg api interface"=w371) -> ("error out"=w367:errorcluster, "rtg api interface out"=w369:refnum<class "NI-RTG Interface.lvclass">)  [unwired: 5 in, 1 out]
              }
            }
            n94 = call-dynamic "Send Target Configuration List - Target Motion.vi"("error in"=w348, "target motion parameters"="Target Motion Parameters", "device index (0)"=w353, "rtg api interface"=w352) -> ("error out"=w350:errorcluster, "rtg api interface out"=w351:refnum<class "NI-RTG Interface.lvclass">)  [unwired: 6 in]
            n95 = case shown="True" w345 {
              tunnel: w351 -> [w359 w364]
              tunnel: [w359 w363] -> w354
              tunnel: w350 -> [w358 w362]
              tunnel: [w358 w361] -> w347
              tunnel: w353 -> [_ w360]
              frame False {
              }
              frame True {
                n96 = call-dynamic "Send Software Trigger.vi"("error in"=w362, "device index (0)"=w360, "NI-RTG Interface in"=w364) -> ("error out"=w361:errorcluster, "NI-RTG Interface out"=w363:refnum<class "NI-RTG Interface.lvclass">)  [unwired: 7 in]
              }
            }
          }
          event "send sw trigger": Value Change {
            # "23"
            n97 = event-data() -> ()  [unwired: 1 in, 1 out]
            n98 = call-dynamic "Send Software Trigger.vi"("error in"=w374, "device index (0)"=w376, "NI-RTG Interface in"=w378) -> ("error out"=w373:errorcluster, "NI-RTG Interface out"=w377:refnum<class "NI-RTG Interface.lvclass">)  [unwired: 7 in]
          }
          event "set hardware trigger": Value Change {
            # "24"
            n99 = event-data() -> ("CtlRef"=w387:refnum<vi>)  [unwired: 1 in]
            n100 = property class="Bool (strict)"(reference=w387, "Value"=FALSE) -> ()  [unwired: 1 in, 2 out]
            n101 = local read "RTG State"() -> (w381:T1)
            n102 = case shown="Default" w381 {
              tunnel: [w390 w396] -> w385
              tunnel: w384 -> [w390 w395]
              tunnel: w383 -> [w389 w392]
              tunnel: w382 -> [_ w394]
              tunnel: [w389 w391] -> w379
              frame "Active" {
                n103 = One Button Dialog(message="Cannot set the trigger while Active.\nStop the RTG and then set the new trigger.") -> ()  [unwired: 1 in, 1 out]
              }
              frame Default {
                n104 = call-dynamic "Set Hardware Trigger.vi"("error in"=w392, "hardware trigger"="Hardware Trigger", "device index (0)"=w394, "rtg api interface"=w395) -> ("error out"=w391:errorcluster, "rtg api interface out"=w396:refnum<class "NI-RTG Interface.lvclass">)  [unwired: 6 in]
              }
            }
          }
          event "start rtg": Value Change {
            # "25"
            n105 = event-data() -> ()  [unwired: 1 in, 1 out]
            n106 = call-dynamic "Start.vi"("error in"=w398, "rtg api interface"=w401) -> ("error out"=w397:errorcluster, "rtg api interface out"=w400:refnum<class "NI-RTG Interface.lvclass">)  [unwired: 8 in]
          }
          event "stop rtg": Value Change {
            # "26"
            # "The Stop is also used to end any current file transfer or target motion operation in progress."
            n107 = event-data() -> ()  [unwired: 1 in, 3 out]
            n108 = call-dynamic "Stop.vi"("error in"=w403, "rtg api interface"=w406) -> ("error out"=w402:errorcluster, "rtg api interface out"=w405:refnum<class "NI-RTG Interface.lvclass">)  [unwired: 8 in]
          }
        }
        n109 = call-dynamic "Get RTG Status.vi"("error in"=w229, "rtg api interface"=w238) -> ("error out"=w236:errorcluster, "rtg status"=w231:string, "state"=w235:T1, "rtg api interface out"=w237:refnum<class "NI-RTG Interface.lvclass">)  [unwired: 6 in]
        n110 = Compound Arithmetic op=OR(w229, w240) -> (w230:bool)
        n111 = local write "RTG State"(w235) -> ()
        n112 = local write "RTG Status"(w231) -> ()
      }
    }
    frame #10 {
      # "31"
      # "30"
      # "28. Stop RTG\n29. Close Coprocessor Resources\n30. Close RTG\n31. Destroy RTG"
      # "28"
      # "Stop RTG, Close Hardware Resouces, and Destroy NI-RTG Object"
      n113 = call-dynamic "Stop.vi"("error in"=w409, "rtg api interface"=w415) -> ("error out"=w408:errorcluster, "rtg api interface out"=w414:refnum<class "NI-RTG Interface.lvclass">)  [unwired: 8 in]
      n114 = for {
        tunnel: w410 -> [w418] mode=indexing
        shift-right: [w416] -> w407
        shift-left: w408 -> [w417]
        # "29"
        n115 = call-dynamic "Close.vi"("error in"=w417, "rtg coprocessor link interface"=w418) -> ("error out"=w416:errorcluster)  [unwired: 9 in]
      }
      n116 = call-dynamic "Close.vi"("error in"=w407, "rtg api interface"=w414) -> ("error out"=w413:errorcluster, "rtg api interface out"=w411:refnum<class "NI-RTG Interface.lvclass">)  [unwired: 8 in]
      n117 = call-dynamic "Destroy.vi"("error in"=w413, "NI-RTG Interface in"=w411) -> ("error out"=→"Error Out":errorcluster)  [unwired: 9 in]
    }
  }
